vi "CleanUp.vi"(8 "error in (no error)":errorcluster, 11 "Object in":refnum<class "Leaf.lvclass">) -> (0 "error out":errorcluster, 3 "object out":refnum<class "Leaf.lvclass">)   [LabVIEW 2019, in "Leaf.lvclass"]
uses:
  Leaf.lvclass
  Sub_class/Sub.lvclass
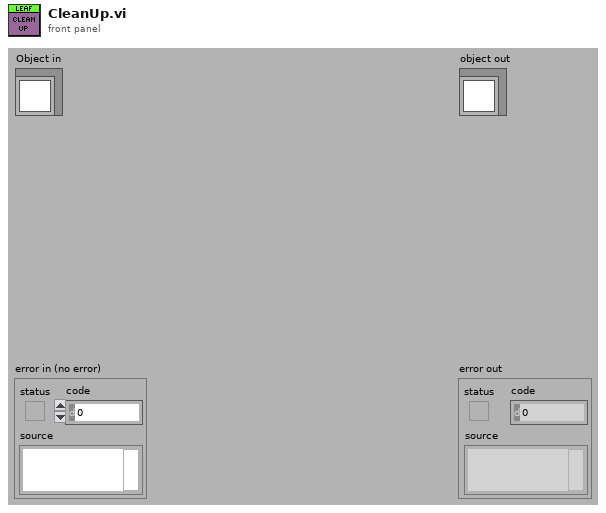
[diagram p1: front panel]
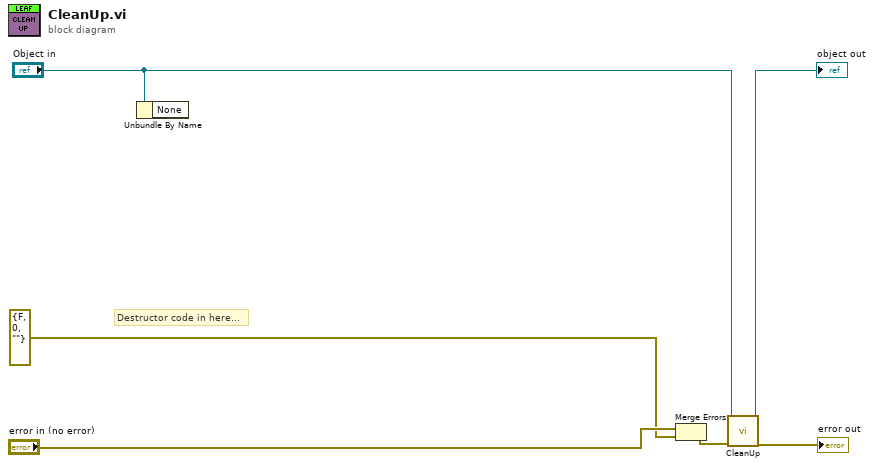
[diagram p0: block diagram]
diagram:
  # "Destructor code in here..."
  n1 = Unbundle By Name("Object in") -> ()  [unwired: 1 out]
  n2 = Merge Errors("error in (no error)", errorcluster {"status"=FALSE, "code"=0, "source"=""} ("error in (no error)")) -> (w2:errorcluster)
  n3 = call-parent "CleanUp.vi"("error in (no error)"=w2, "Object in"="Object in") -> ("error out"=→"error out":errorcluster, "object out"=→"object out":refnum<class "Leaf.lvclass">)  [unwired: 8 in]
